vi "Write scopes.vi"(8 "error in (no error)":errorcluster, 10 "scopes":string[](array[string]), 11 "Oauth2 in":refnum<class "Oauth2.lvclass">) -> (0 "error out":errorcluster, 3 "Oauth2 out":refnum<class "Oauth2.lvclass">)   [LabVIEW 2013, in "Oauth2.lvclass"]
uses:
  Oauth2.lvclass
  Oauth2.lvclass/Oauth2.ctl
  OAuthToken/OAuth2 Token Element -- enum.ctl
  OAuthToken/OAuthAccessToken.lvclass
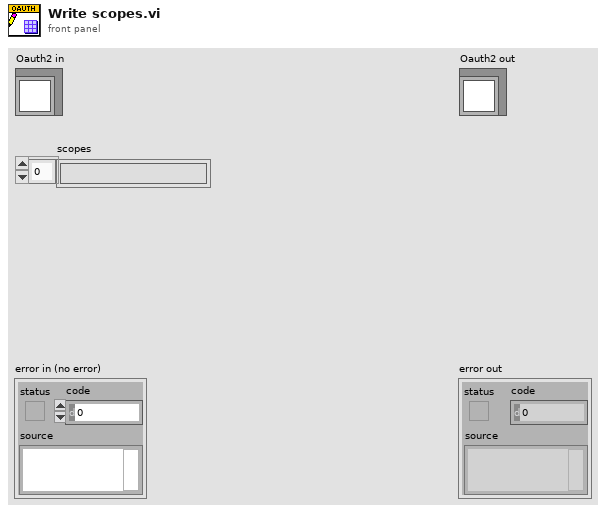
[diagram p1: front panel]
types:
  T1 = typedef "OAuthAccessToken.lvclass/OAuth2 Token Element -- enum.ctl" = enum16{"client_id", "client_secret", "response_type", "scope", "redirect_uri", "error", "error_description", "error_uri", "grant_type", "code", "access_token", "token_type", "expires_in", "username", "password", "refresh_token", "endpoint element"}
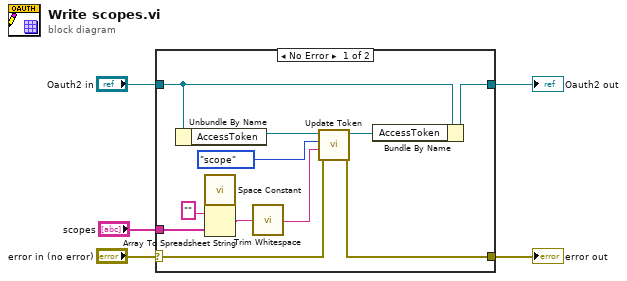
[diagram p0: block diagram]
diagram:
  n1 = case shown="No Error" "error in (no error)" {
    selector: "error in (no error)" -> [w13 w18]
    tunnel: [w12 w18] -> w3
    tunnel: [w6 w19] -> w4
    tunnel: "Oauth2 in" -> [w7 w19]
    tunnel: "scopes" -> [w11 _]
    frame No Error {
      n2 = Unbundle By Name(w7) -> ("AccessToken"=w15:refnum<class "OAuthAccessToken.lvclass">)
      n3 = call <vilib>:"Space Constant.vi"() -> ("String"=w17:string)
      n4 = Array To Spreadsheet String(delimiter (Tab)=w17, array=w11, 3:"" ("format string")) -> (spreadsheet string=w10:string)
      n5 = call <vilib>:"Trim Whitespace.vi"("string"=w10) -> ("trimmed string"=w9:string)  [unwired: 1 in]
      n6 = call "Update Token.vi"("error in (no error)"=w13, "Value"=w9, "Token element"=OAuth2_Token_Element_--_enum."scope", "OAuthAccessToken in"=w15) -> ("error out"=w12:errorcluster, "OAuthAccessToken out"=w8:refnum<class "OAuthAccessToken.lvclass">)  [unwired: 6 in]
      n7 = Bundle By Name(cluster=w7, "AccessToken"=w8) -> (w6:refnum<class "Oauth2.lvclass">)
    }
    frame Error {
    }
  }
  "error out" <- w3
  "Oauth2 out" <- w4
